vi "method parameters.disable empty elements.vi"(0 "control ref":refnum<vi>, 2 "Data In":T1, 4 "State":T2, 5 "error in (no error)":errorcluster) -> (19 "error out":errorcluster)   [LabVIEW 2014, in "method parameters.xctl"]
uses:
  method parameters.xctl
  method parameters.State.ctl
  method parameters.Data.ctl
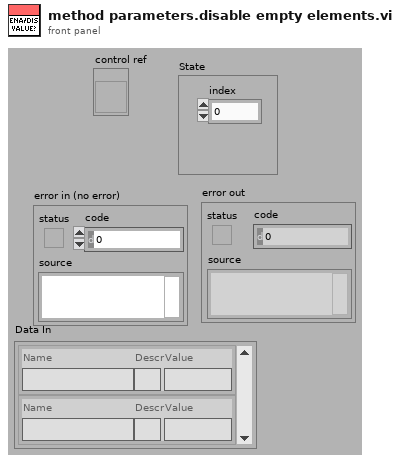
[diagram p1: front panel]
types:
  T1 = typedef "method parameters.xctl/method parameters.Data.ctl" = cluster{"Name":string, "Descr":string, "Value":string}[]
  T2 = typedef "method parameters.xctl/method parameters.State.ctl" = cluster{"index":i32}
  T3 = enum8{"Enabled", "Disabled", "Disabled and Grayed Out"}
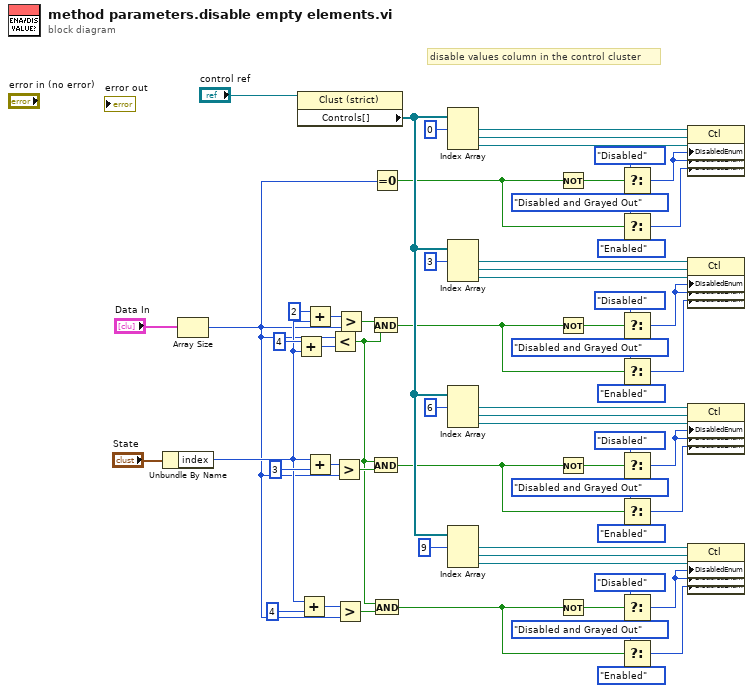
[diagram p0: block diagram]
diagram:
  w14 = T3."Disabled and Grayed Out" ("Disabled")
  w23 = T3."Disabled and Grayed Out" ("Disabled")
  w34 = T3."Disabled and Grayed Out" ("Disabled")
  w43 = T3."Disabled and Grayed Out" ("Disabled")
  # "disable values column in the control cluster"
  n1 = Unbundle By Name("State") -> ("index"=w3:i32)
  n2 = Array Size(array="Data In") -> (size(s)=w1:i32)
  n3 = Add(x=4, y=w3) -> (x+y=w55:i32)
  n4 = property class="Clust (strict)"(reference="control ref") -> ("Controls[]"=w62:refnum<vi>[])  [unwired: 1 in, 2 out]
  n5 = Add(x=w3, y=4) -> (x+y=w51:i32)
  n6 = Add(x=2, y=w3) -> (x+y=w54:i32)
  n7 = Add(x=w3, y=3) -> (x+y=w52:i32)
  n8 = Less?(x=w1, y=w55) -> (x < y?=w57:bool)
  n9 = Greater?(x=w52, y=w1) -> (0:w59:bool)
  n10 = Greater?(x=w51, y=w1) -> (0:w58:bool)
  n11 = Greater?(x=w54, y=w1) -> (0:w61:bool)
  n12 = And(x=w61, y=w57) -> (x .and. y?=w31:bool)
  n13 = And(x=w57, y=w59) -> (x .and. y?=w21:bool)
  n14 = Equal To 0?(x=w1) -> (x = 0?=w38:bool)
  n15 = And(x=w57, y=w58) -> (x .and. y?=w11:bool)
  n16 = Index Array(array=w62, index #1=0) -> (element #1=w42:refnum<vi>, element #2=w41:refnum<vi>, element #3=w40:refnum<vi>)  [unwired: 2 in]
  n17 = Index Array(array=w62, index #1=3) -> (element #1=w30:refnum<vi>, element #2=w29:refnum<vi>, element #3=w28:refnum<vi>)  [unwired: 2 in]
  n18 = Index Array(array=w62, index #1=6) -> (element #1=w20:refnum<vi>, element #2=w18:refnum<vi>, element #3=w17:refnum<vi>)  [unwired: 2 in]
  n19 = Index Array(array=w62, index #1=9) -> (element #1=w10:refnum<vi>, element #2=w9:refnum<vi>, element #3=w6:refnum<vi>)  [unwired: 2 in]
  n20 = Not(x=w38) -> (.not. x?=w39:bool)
  n21 = Not(x=w31) -> (.not. x?=w35:bool)
  n22 = Not(x=w21) -> (.not. x?=w22:bool)
  n23 = Not(x=w11) -> (.not. x?=w15:bool)
  n24 = Select(t=T3."Disabled" ("Disabled"), s=w39, f=w43) -> (s? t:f=w37:T3)
  n25 = Select(t=w43, s=w38, f=T3."Enabled" ("Disabled")) -> (s? t:f=w36:T3)
  n26 = Select(t=T3."Disabled" ("Disabled"), s=w35, f=w34) -> (s? t:f=w27:T3)
  n27 = Select(t=w34, s=w31, f=T3."Enabled" ("Disabled")) -> (s? t:f=w26:T3)
  n28 = Select(t=T3."Disabled" ("Disabled"), s=w22, f=w23) -> (s? t:f=w19:T3)
  n29 = Select(t=w23, s=w21, f=T3."Enabled" ("Disabled")) -> (s? t:f=w16:T3)
  n30 = Select(t=T3."Disabled" ("Disabled"), s=w15, f=w14) -> (s? t:f=w8:T3)
  n31 = Select(t=w14, s=w11, f=T3."Enabled" ("Disabled")) -> (s? t:f=w7:T3)
  n32 = property class="Ctl"(reference=w42, "DisabledEnum"=w37) -> ()  [unwired: 1 in, 2 out]
  n33 = property class="Ctl"(reference=w41, "DisabledEnum"=w37) -> ()  [unwired: 1 in, 2 out]
  n34 = property class="Ctl"(reference=w40, "DisabledEnum"=w36) -> ()  [unwired: 1 in, 2 out]
  n35 = property class="Ctl"(reference=w30, "DisabledEnum"=w27) -> ()  [unwired: 1 in, 2 out]
  n36 = property class="Ctl"(reference=w29, "DisabledEnum"=w27) -> ()  [unwired: 1 in, 2 out]
  n37 = property class="Ctl"(reference=w28, "DisabledEnum"=w26) -> ()  [unwired: 1 in, 2 out]
  n38 = property class="Ctl"(reference=w20, "DisabledEnum"=w19) -> ()  [unwired: 1 in, 2 out]
  n39 = property class="Ctl"(reference=w18, "DisabledEnum"=w19) -> ()  [unwired: 1 in, 2 out]
  n40 = property class="Ctl"(reference=w17, "DisabledEnum"=w16) -> ()  [unwired: 1 in, 2 out]
  n41 = property class="Ctl"(reference=w10, "DisabledEnum"=w8) -> ()  [unwired: 1 in, 2 out]
  n42 = property class="Ctl"(reference=w9, "DisabledEnum"=w8) -> ()  [unwired: 1 in, 2 out]
  n43 = property class="Ctl"(reference=w6, "DisabledEnum"=w7) -> ()  [unwired: 1 in, 2 out]
